vi "4feladat.vi"() -> ()   [LabVIEW 2016]
panel:
  out "Rész-számítás":dbl
  out "Futási sebesség":dbl
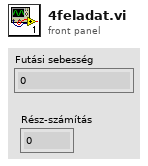
[diagram p1: front panel]
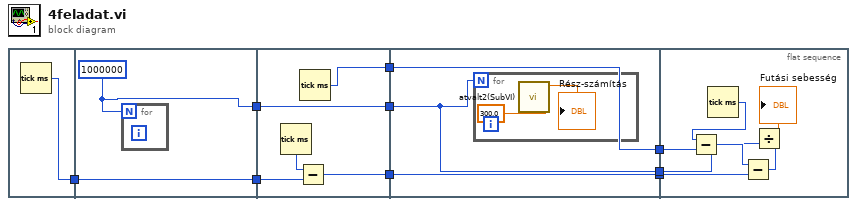
[diagram p0: block diagram]
diagram:
  n1 = flat-sequence {
    tunnel: [w10] -> w6
    tunnel: [w12] -> w7
    tunnel: w6 -> [w12]
    tunnel: [w11] -> w2
    tunnel: [w17] -> w8
    tunnel: w7 -> [w16]
    tunnel: [w14] -> w4
    tunnel: [w13] -> w3
    tunnel: w2 -> [w13]
    tunnel: [w20] -> w9
    tunnel: w8 -> [w20]
    tunnel: [w19] -> w5
    tunnel: w4 -> [w19]
    tunnel: w3 -> [w18]
    tunnel: [w18] -> w1
    tunnel: w9 -> [w28]
    tunnel: w5 -> [w26]
    tunnel: w1 -> [w24]
    frame #0 {
      n2 = Tick Count (ms)() -> (millisecond timer value=w10:u32)
    }
    frame #1 {
      w11 = 1000000
      n3 = for {
        N: w11 -> [_]
      }
    }
    frame #2 {
      n4 = Tick Count (ms)() -> (millisecond timer value=w15:u32)
      n5 = Subtract(x=w15, y=w16) -> (x-y=w14:u32)
      n6 = Tick Count (ms)() -> (millisecond timer value=w17:u32)
    }
    frame #3 {
      n7 = for {
        N: w18 -> [_]
        n8 = call "atvalt2(SubVI).vi"("Numeric in"=300.0) -> ("Numeric out"=→"Rész-számítás":dbl)  [unwired: 10 in]
      }
    }
    frame #4 {
      n9 = Tick Count (ms)() -> (millisecond timer value=w29:u32)
      n10 = Subtract(x=w29, y=w28) -> (x-y=w27:u32)
      n11 = Subtract(x=w27, y=w26) -> (x-y=w25:u32)
      n12 = Divide(x=w25, y=w24) -> (x/y=→"Futási sebesség":dbl)
    }
  }
